vi "3D-SplitPosString.vi"(8 "索引":i32, 11 "input pos array":string[][](array[string])) -> (0 "Y pos":i32, 1 "Y pos":string, 2 "X pos":string, 3 "X pos":i32)   [LabVIEW 2015]
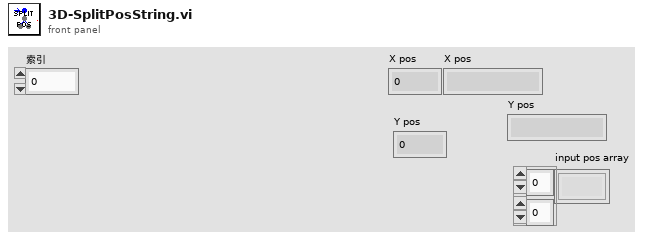
[diagram p1: front panel]
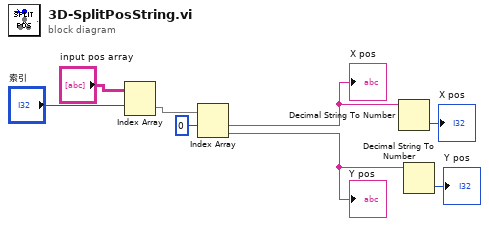
[diagram p0: block diagram]
diagram:
  n1 = Index Array(array="input pos array", index (row)="索引") -> (element=w4:string[])  [unwired: 1 in]
  n2 = Index Array(array=w4, index #1=0 ("索引")) -> (element #1=w2:string, element #2=w1:string)  [unwired: 1 in]
  "X pos" <- w2
  "Y pos" <- w1
  n3 = Decimal String To Number(string=w2) -> (number=→"X pos":i32)  [unwired: 2 in, 1 out]
  n4 = Decimal String To Number(string=w1) -> (number=→"Y pos":i32)  [unwired: 2 in, 1 out]
